vi "SettingVariable.vi"() -> ()   [LabVIEW 2020]
panel:
  in  "voltage outputs":T1(array[cluster]) {"voltage lower" min=-10 max=10; "voltage upper" min=-10 max=10}
  in  "source":dbl
  in  "lifetime":dbl
  in  "lambda":dbl[](array[numeric])
  in  "beta":dbl[](array[numeric])
  in  "DRWM path 2":path
  in  "DRWM path 1":path
  in  "data path":path
  in  "current inputs":cluster{"name":string, "switch":bool}[](array[cluster])
  in  "deltaT":dbl
  in  "voltage inputs":T2(array[cluster]) {"scale" items=["计数通量log", "电压通量", "电流通量log", "棒位", "温度", "P2参数", "硼浓度"]; "voltage lower" min=-10 max=10; "voltage upper" min=-10 max=10}
  out "IP":string
  out "port":u16
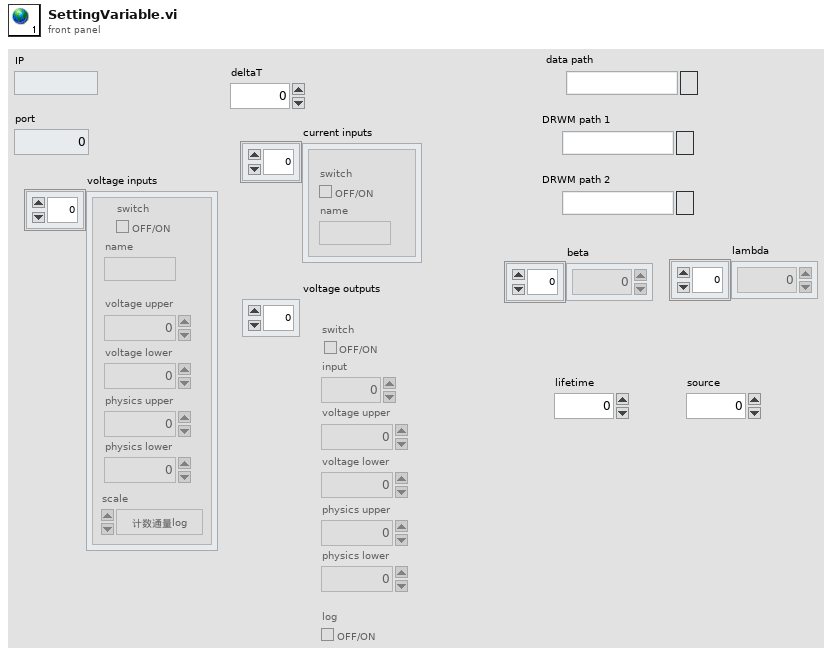
[diagram p1: front panel]
types:
  T1 = cluster{"switch":bool, "voltage upper":i32, "voltage lower":i32, "physics upper":dbl, "physics lower":dbl, "input":u16, "log":bool}[]
  T2 = cluster{"switch":bool, "name":string, "voltage upper":i32, "voltage lower":i32, "physics upper":dbl, "physics lower":dbl, "scale":u16}[]
diagram:
